vi "LineColorStart.vi"(7 "TestBoxs:":refnum<vi>, 8 "error in":errorcluster, 9 "DisplayRow":i32=17, 10 "ReadRow":i32, 11 "Color Box":u32(colorbox)=16776960) -> (0 "error out":errorcluster, 4 "Time":u32, 5 "TestBoxs:":refnum<vi>, 6 "ReadRow":i32)   [LabVIEW 2013]
uses:
  <vilib>/Utility/miscctls.llb/LVRowAndColumnTypeDef.ctl
  Control/Read&Write.ctl
panel:
  in  "Blink?":bool=TRUE
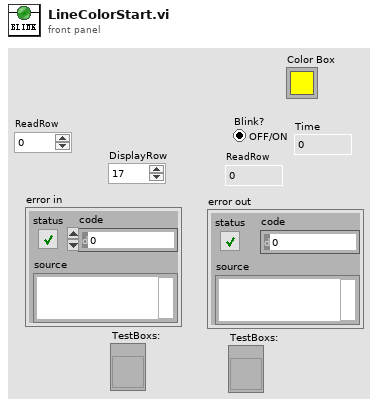
[diagram p1: front panel]
types:
  T1 = typedef "Read&Write.ctl" = enum16{"Read", "Write"}
  T2 = typedef "LVRowAndColumnTypeDef.ctl" = cluster{"Row":i32, "Column":i32}
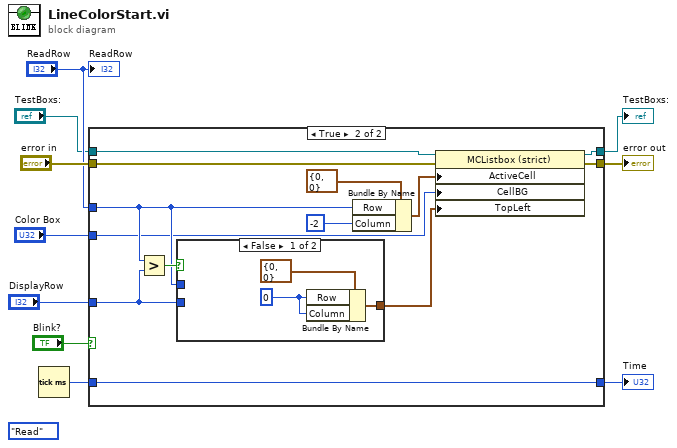
[diagram p0: block diagram]
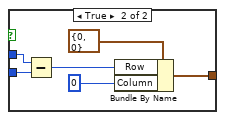
[diagram p3: hidden frame]
diagram:
  (unwired) Read&Write."Read" ("Enum-Read/Write")
  n1 = Tick Count (ms)() -> (millisecond timer value=w4:u32)
  n2 = case shown="True" "Blink?" {
    tunnel: "TestBoxs:" -> [w13 w26]
    tunnel: [w13 w25] -> w5
    tunnel: "DisplayRow" -> [_ w19]
    tunnel: "ReadRow" -> [_ w18]
    tunnel: "Color Box" -> [_ w17]
    tunnel: "error in" -> [w12 w16]
    tunnel: [w12 w15] -> w6
    tunnel: [w11 w14] -> w3
    tunnel: w4 -> [w11 w14]
    frame False {
    }
    frame True {
      n3 = Greater?(x=w18, y=w19) -> (0:w21:bool)
      n4 = case shown="False" w21 {
        tunnel: w18 -> [_ w33]
        tunnel: [w28 w31] -> w20
        tunnel: w19 -> [_ w30]
        frame False {
          w27 = 0 ("Column")
          n5 = Bundle By Name(cluster=T2 {"Row"=0, "Column"=0} ("Active Cell"), "Row"=w27, "Column"=w27) -> (w28:T2)
        }
        frame True {
          n6 = Subtract(x=w33, y=w30) -> (x-y=w32:i32)
          n7 = Bundle By Name(cluster=T2 {"Row"=0, "Column"=0} ("Active Cell"), "Row"=w32, "Column"=0) -> (w31:T2)
        }
      }
      n8 = Bundle By Name(cluster=T2 {"Row"=0, "Column"=0} ("Active Cell"), "Row"=w18, "Column"=-2) -> (w22:T2)
      n9 = property on="Property Node" class="MCListbox (strict)"(reference=w26, error in=w16, "ActiveCell"=w22, "CellBG"=w17, "TopLeft"=w20) -> (reference out=w25:refnum<vi>, error out=w15:errorcluster)
    }
  }
  "error out" <- w6
  "Time" <- w3
  "TestBoxs:" <- w5
  "ReadRow" <- "ReadRow"
